vi "Timing Engine.vi"(8 "error in (no error)":errorcluster, 10 "Time Limit (sec)":dbl, 11 "Timing Cmd In":T1) -> (0 "error out":errorcluster, 2 "Done?":bool, 3 "Elaspsed TIme (sec)":u32)   [LabVIEW 2018, in "Timing.lvlib" / "Timing Action Engine.lvlib"]
doc: "Timing Engine provides functionality to Main Vi"
uses:
  Timing Action Engine.lvlib
  TimingCmd Enum.ctl
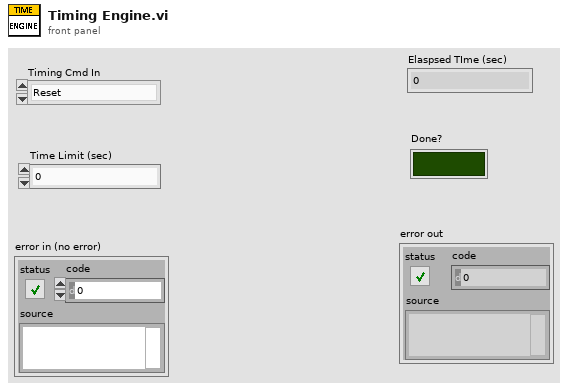
[diagram p1: front panel]
types:
  T1 = typedef "Timing.lvlib/Timing Action Engine.lvlib/TimingCmd Enum.ctl" = enum16{"Reset", "Pause", "Read Time"}
  T2 = typedef "Timing.lvlib/Timing Action Engine.lvlib/Timing Params.ctl" = cluster{"Tick Count (msec)":T3, "Elaspsed TIme (sec)":dbl}
  T3 = typedef "Timing.lvlib/Timing Action Engine.lvlib/TickCount.ctl" = u32
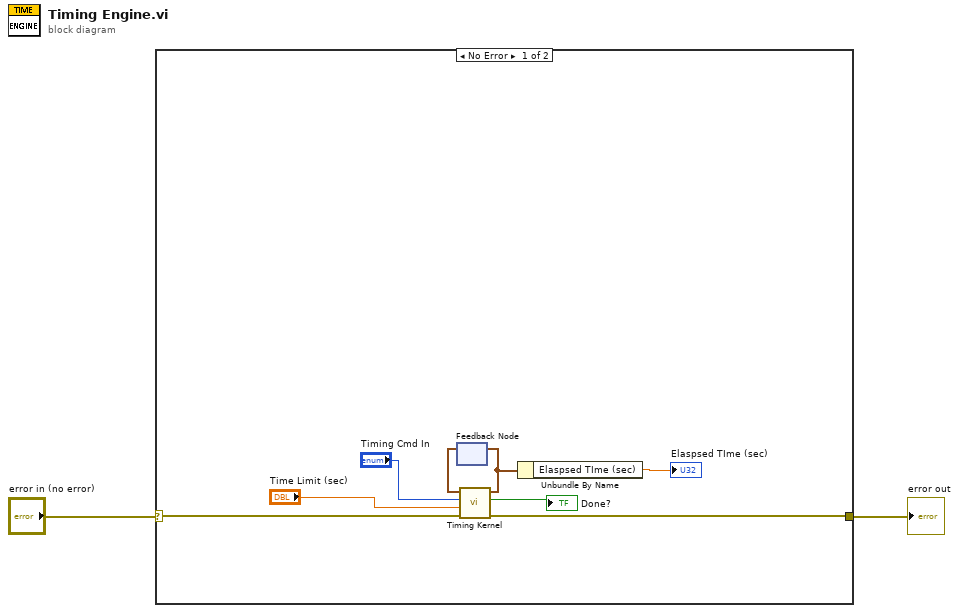
[diagram p0: block diagram]
diagram:
  n1 = case shown="No Error" "error in (no error)" {
    selector: "error in (no error)" -> [w9 w11]
    tunnel: [w8 w11] -> w1
    frame No Error {
      n2 = feedback #1() -> (w5:T2)  [unwired: 1 in]
      n3 = call "Timing Kernel.vi"("error in (no error)"=w9, "Time Limit (sec)"="Time Limit (sec)", "Timing Cmd In"="Timing Cmd In", "Timing params in"=w5) -> ("error out"=w8:errorcluster, "Done?"=→"Done?":bool, "Timing params Out"=w4:T2)  [unwired: 5 in]
      n4 = feedback-in #1(w4) -> ()
      n5 = Unbundle By Name(w4) -> ("Elaspsed TIme (sec)"=→"Elaspsed TIme (sec)":dbl)
    }
    frame Error {
    }
  }
  "error out" <- w1
